vi "u_sat.vi"(2 "error in (no error)":errorcluster, 3 "u":dbl) -> (0 "error out":errorcluster, 1 "u_sat":dbl)   [LabVIEW 2019]
panel:
  out "max":dbl
  out "min":dbl
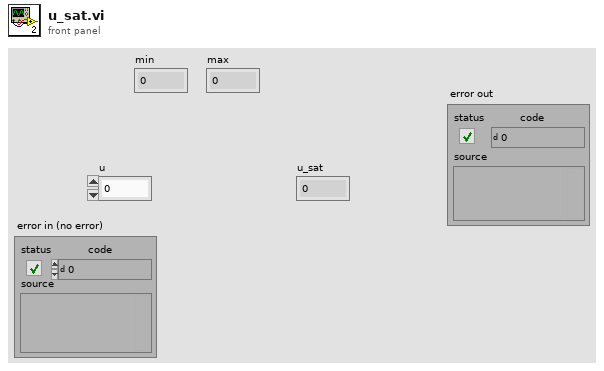
[diagram p1: front panel]
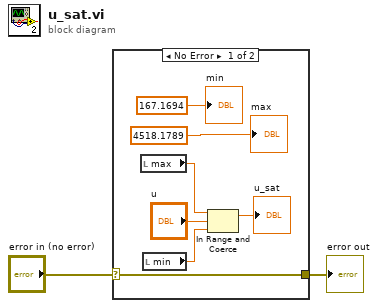
[diagram p0: block diagram]
diagram:
  n1 = case shown="No Error" "error in (no error)" {
    selector: "error in (no error)" -> [w3 w10]
    tunnel: [w3 w10] -> w1
    frame No Error {
      n2 = local read "max"() -> (w5:dbl)
      n3 = local read "min"() -> (w6:dbl)
      n4 = In Range and Coerce(upper limit=w5, x="u", lower limit=w6) -> (coerced(x)=→"u_sat":dbl)  [unwired: 1 out]
      "min" <- 167.1694 ("min")
      "max" <- 4518.1789 ("max")
    }
    frame Error {
    }
  }
  "error out" <- w1
